vi "Global 1.vi"() -> ()   [LabVIEW 2013]
uses:
  <userlib>/KNR OS 3.0 LabVIEW Toolkit/Type Definition/DC Motor Port.ctl
panel:
  in  "C区偏差值":dbl=24.0
  in  "障碍偏差绝对值":dbl=31.0
  in  "AE距离":dbl=30.0
  in  "弹射速度":dbl=-100.0
  in  "DC3弹射":T1=6 items=["DS1"=4, "DS2"=5, "DS3"=6, "DS4"=7]
  in  "角度范围":dbl=42.0
  in  "击球偏差":dbl=-22.0
  in  "挖杆挖起":dbl=700.0
  in  "挖杆下潜":dbl=1750.0
  in  "挖杆准备":dbl=2500.0
  in  "调整慢速":dbl=7.0
  in  "前进速度":dbl=13.0
  in  "转弯速度":dbl=10.0
  in  "光感阈值":i32=1800
  in  "AB右转弯":dbl=90.0
  in  "买菜左转弯":dbl=90.0
  in  "取第3个球距离":dbl=-11.5
  in  "取第2个球距离":dbl=-16.0
  in  "超声波阈值":i32=17
  in  "出门左转弯":dbl=-89.0
  in  "取第1个球距离":dbl=-5.6
  in  "买菜距离":dbl=10.0
  out "走到警示线":dbl
  in  "DC1左轮":T1=4 items=["DS1"=4, "DS2"=5, "DS3"=6, "DS4"=7]
  in  "DC2右轮":T1=5 items=["DS1"=4, "DS2"=5, "DS3"=6, "DS4"=7]
  in  "轮直径d":dbl=9.5
  in  "车直径D":dbl=28.5
  out "转弯后到取球距离":dbl
  in  "出门微调":dbl=1.3
  # "DE去-20 C区-10"
  # "纠正偏差"
  # "出基地后退到光感捕捉到基地的线"
  # "目标与中心点的偏差/640 *角度范围"
  # "右正的话会大一点"
  # "左逆是刚好"
  # "识别"
  # "DE区，right，31\nAB区，left  ，"
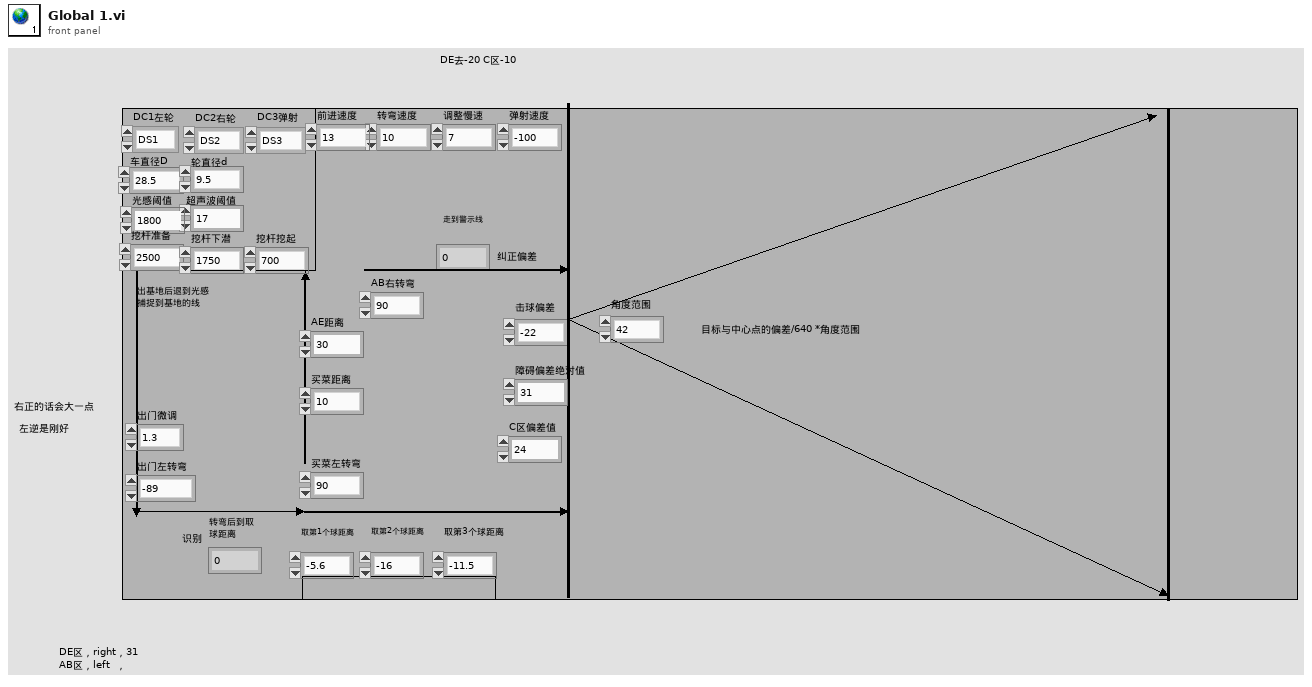
[diagram p1: front panel]
types:
  T1 = typedef "DC Motor Port.ctl" = u16
diagram:
